vi "Test For Square of Color.vi"(8 "color":u32(colorbox)=65535, 9 "column":i16=1, 10 "row":i16=1, 11 "board image":T1) -> (2 "pass?":T2)   [LabVIEW 2018, in "Board Design.lvclass"]
doc: "Check the image for the presence of a square of the given color at the given location."
uses:
  Board Design.lvclass
  Common/Pass Fail Boolean.ctl
  Common/Board Image.ctl
  Assembly Line Input_class/Assembly Line Input.lvclass
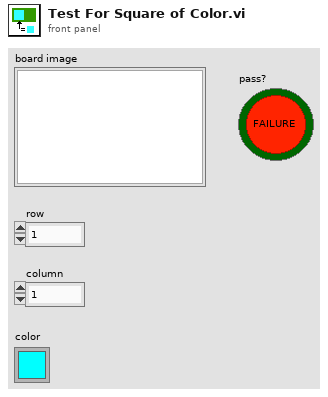
[diagram p1: front panel]
types:
  T1 = typedef "Board Image.ctl" = picture
  T2 = typedef "Pass Fail Boolean.ctl" = bool
  T3 = cluster{"left":i16, "top":i16, "right":i16, "bottom":i16}
  T4 = typedef "imagedata.ctl" = cluster{"image type":i32, "image depth":i32, "image":u8[], "mask":u8[], "colors":u32[], "Rectangle":cluster{"left":i16, "top":i16, "right":i16, "bottom":i16}}
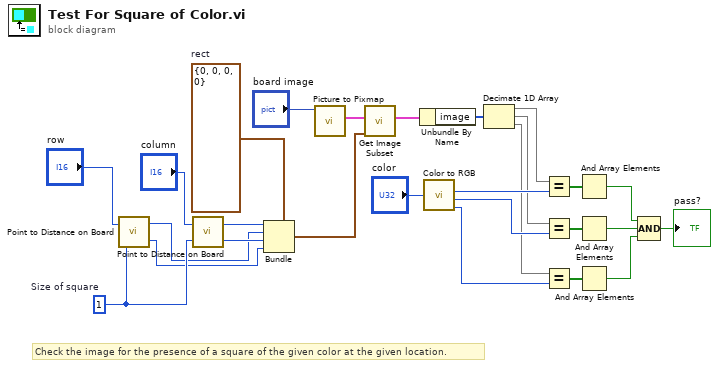
[diagram p0: block diagram]
diagram:
  w22 = T3 {"left"=0, "top"=0, "right"=0, "bottom"=0}  # rect
  w25 = i16 1  # Size of square
  # "Check the image for the presence of a square of the given color at the given location."
  n1 = call "Point to Distance on Board.vi"("Size of square"=w25, "scaled value"="row") -> ("end pixel"=w18:i16, "start pixel"=w19:i16)
  n2 = call "Point to Distance on Board.vi"("Size of square"=w25, "scaled value"="column") -> ("end pixel"=w20:i16, "start pixel"=w21:i16)
  n3 = Bundle(cluster=w22, "left"=w21, "top"=w19, "right"=w20, "bottom"=w18) -> (w17:T3)
  n4 = call <vilib>:"Picture to Pixmap.vi"("picture"="board image") -> ("image data"=w23:T4)  [unwired: 9 in, 1 out]
  n5 = call <vilib>:"Get Image Subset.vi"("subset rect"=w17, "image data"=w23) -> ("image subset"=w16:T4)  [unwired: 4 in, 1 out]
  n6 = Unbundle By Name(w16) -> ("image"=w14:u8[])
  n7 = call <vilib>:"Color to RGB.vi"("Color"="color") -> ("R"=w12:u8, "G"=w10:u8, "B"=w8:u8)  [unwired: 1 out]
  n8 = Decimate 1D Array(w14) -> (w13:u8[], w11:u8[], w9:u8[])
  n9 = Equal?(x=w13, y=w12) -> (x = y?=w7:bool[])
  n10 = Equal?(x=w11, y=w10) -> (x = y?=w6:bool[])
  n11 = Equal?(x=w9, y=w8) -> (x = y?=w5:bool[])
  n12 = And Array Elements(Boolean array=w7) -> (logical AND=w4:bool)
  n13 = And Array Elements(Boolean array=w6) -> (logical AND=w3:bool)
  n14 = And Array Elements(Boolean array=w5) -> (logical AND=w2:bool)
  n15 = Compound Arithmetic op=AND(w4, w3, w2) -> (→"pass?":bool)
